vi "Main.vi"() -> ()   [LabVIEW 2023]
doc: "This template is for the Queued Message Handler design pattern.\n\nThe Event Handling Loop generates messages based on user interface actions.\n\nThe Message Handling Loop processes messages generated by the Event Handling Loop, or by other messages. The messages are string values, so new messages can be added easily to the Message Cases case structure in the Message Handling Loop. Each message cluster can also provide an optional value for Message Data, which is a variant that can be converted to whatever message-specific data is required."
uses:
  <extravilib>/ChannelInstances/Messenger-t'Message Queue.lvlib-Message Cluster.ctl'/Instantiate.vi
  <vilib>/Utility/error.llb/Error Cluster From Error Code.vi
  <extravilib>/ChannelInstances/Event Messenger-bool/))Channel.vi
  <extravilib>/ChannelInstances/Event Messenger-bool/Instantiate.vi
  <vilib>/ErrorRing/Error Ring.xnode
  <extravilib>/ChannelInstances/Event Messenger-bool.lvlib
  support/Message Queue/Message Queue.lvlib
panel:
  out "Loop Iteration Time":u32
  out "Create Data Time":u32
  out "ITER":i32
  out "Intensity Graph":u8[][](graph)
  in  "Start Parallel":bool
  in  "Exit":bool
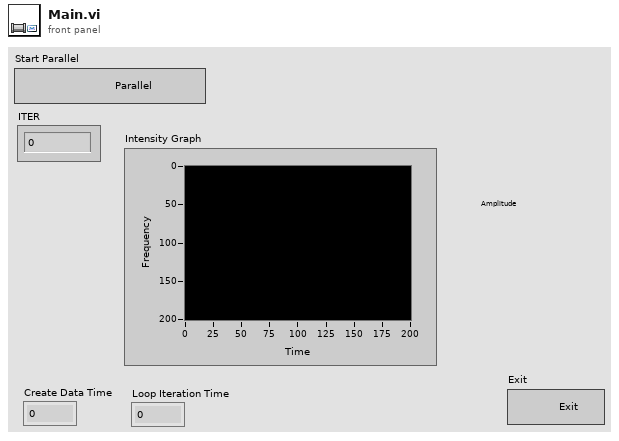
[diagram p1: front panel]
types:
  T1 = typedef "Messenger-t'Message Queue.lvlib-Message Cluster.ctl'.lvlib/))Channel.ctl" = refnum<queue>
  T2 = typedef "Event Messenger-bool.lvlib/))Channel.ctl" = refnum<queue>
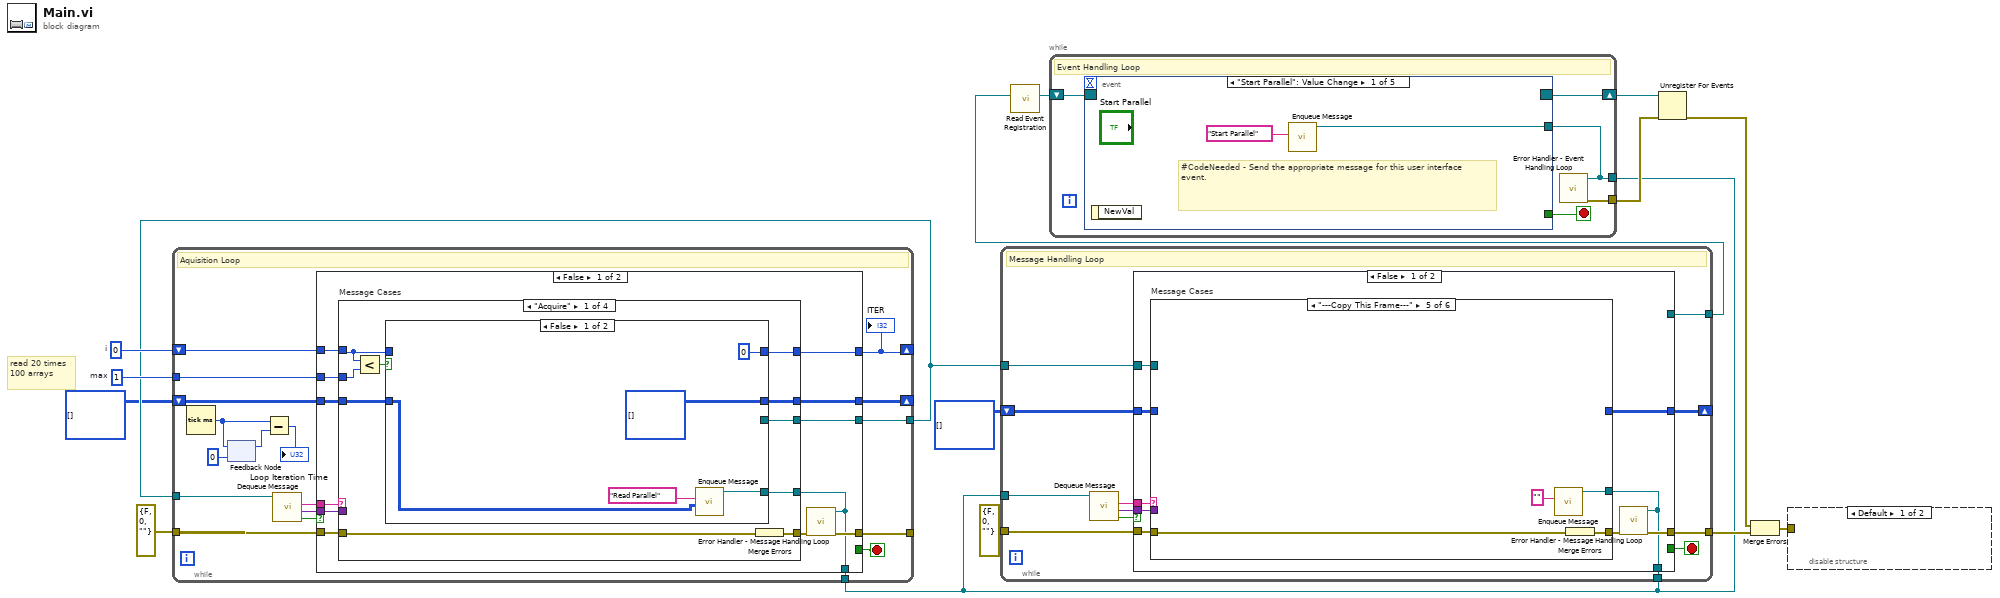
[diagram p0: block diagram]
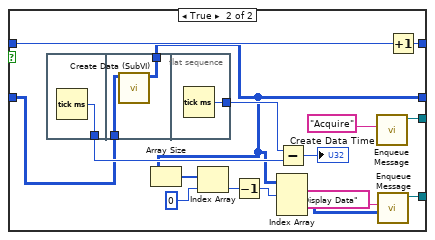
[diagram p2: hidden frame]
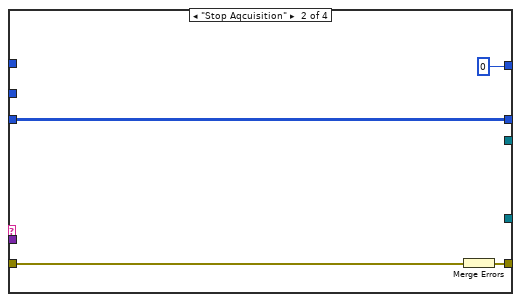
[diagram p3: hidden frame]
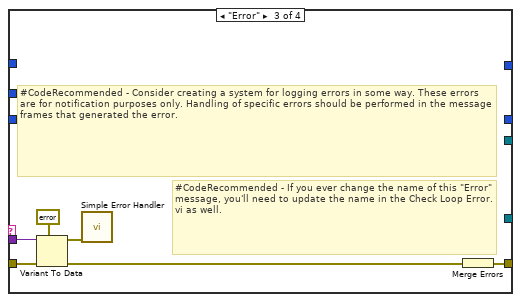
[diagram p4: hidden frame]
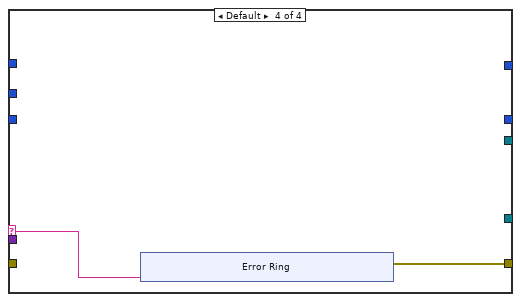
[diagram p5: hidden frame]
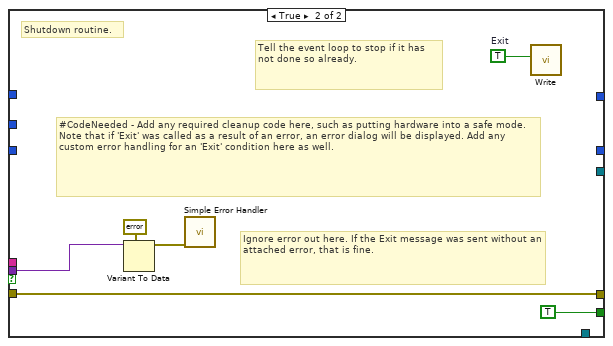
[diagram p6: hidden frame]
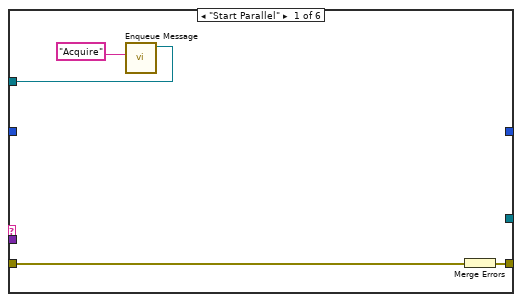
[diagram p7: hidden frame]
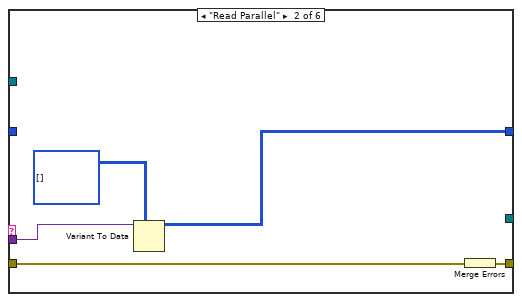
[diagram p8: hidden frame]
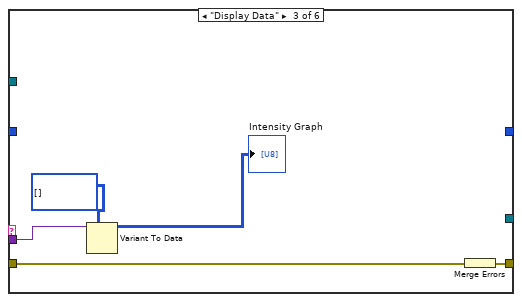
[diagram p9: hidden frame]
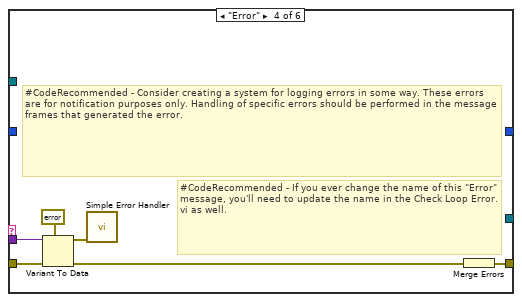
[diagram p10: hidden frame]
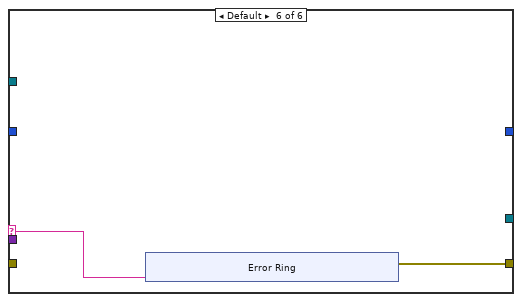
[diagram p11: hidden frame]
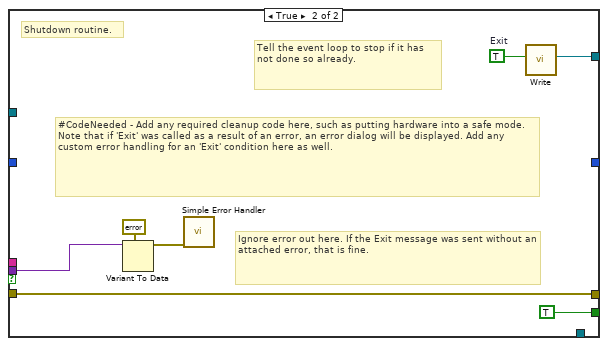
[diagram p12: hidden frame]
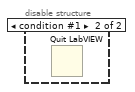
[diagram p13: hidden frame]
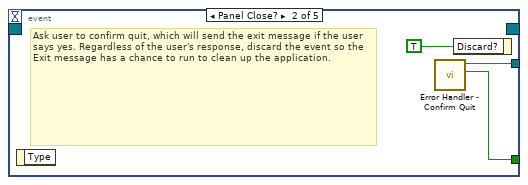
[diagram p14: hidden frame]
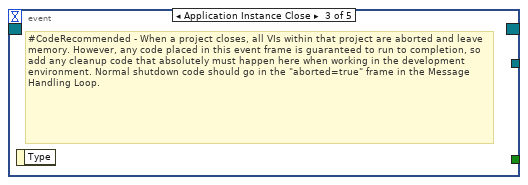
[diagram p15: hidden frame]
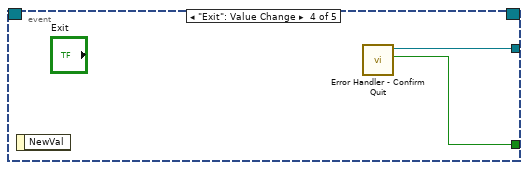
[diagram p16: hidden frame]
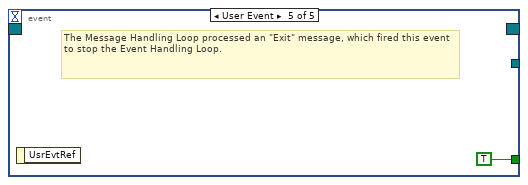
[diagram p17: hidden frame]
diagram:
  w4 = 0  # i
  w5 = 1  # max
  # "read 20 times\n100 arrays"
  n1 = while {
    tunnel: [w32] -> _
    tunnel: w3 -> [w29]
    tunnel: errorcluster {"status"=FALSE, "code"=0, "source"=""} ("error IO") -> [w31]
    tunnel: [w30] -> w6
    tunnel: w5 -> [w25]
    shift-right: [w23] -> _
    shift-left: w4 -> [w24]
    tunnel: [w22] -> w3
    shift-right: [w17] -> _
    shift-left: u8[][][] [] ("element") -> [w16]
    stop <- w33 stop-if-true
    # "Aquisition Loop"
    n2 = Tick Count (ms)() -> (millisecond timer value=w19:u32)
    n3 = feedback-in #1(w19) -> ()
    n4 = feedback #1(u32 0 ("millisecond timer value")) -> (w20:u32)
    n5 = Subtract(x=w19, y=w20) -> (x-y=→"Loop Iteration Time":u32)
    n6 = call "Dequeue Message.vi"("channel"=w29) -> ("channel aborted"=w26:bool, "message data"=w27:variant, "message"=w28:string)  [unwired: 8 in]
    n7 = case shown="False" w26 {
      tunnel: [_ TRUE] -> w33
      tunnel: [w45 w104] -> w32
      tunnel: w28 -> [w43 _]
      tunnel: w27 -> [w42 w101]
      tunnel: w31 -> [w41 w104]
      tunnel: [w40 _] -> w30
      tunnel: w25 -> [w39 _]
      tunnel: w24 -> [w38 _]
      tunnel: [w37 _] -> w23
      tunnel: [w36 _] -> w22
      tunnel: w16 -> [w35 _]
      tunnel: [w34 _] -> w17
      frame False {
        n8 = case "Message Cases" shown="\"Acquire\"" w43 {
          selector: w43 -> [_ _ _ w91]
          tunnel: w41 -> [w54 w83 w90 _]
          tunnel: [w55 w84 w85 w92] -> w44
          tunnel: w42 -> [_ _ w89 _]
          tunnel: [w53 _ _ _] -> w40
          tunnel: w39 -> [w49 _ _ _]
          tunnel: w38 -> [w50 _ _ _]
          tunnel: [w52 0 _ _] -> w37
          tunnel: [w48 _ _ _] -> w36
          tunnel: w35 -> [w47 w81 _ _]
          tunnel: [w46 w81 _ _] -> w34
          frame "Acquire" {
            # "Something - Replace this message with functionality for your own application."
            n9 = Less?(x=w50, y=w49) -> (x < y?=w51:bool)
            n10 = case shown="False" w51 {
              tunnel: [w58 w76] -> w53
              tunnel: [0 w74] -> w52
              tunnel: w50 -> [_ w73]
              tunnel: [_ w71] -> w48
              tunnel: w47 -> [w56 w67]
              tunnel: [u8[][][] [] ("element") w62] -> w46
              frame False {
                n11 = call "Enqueue Message.vi"("data (empty)"=w56, "message"="Read Parallel") -> ("channel"=w58:T1)  [unwired: 9 in]
              }
              frame True {
                n12 = flat-sequence {
                  tunnel: [w77] -> w69
                  tunnel: w67 -> [w78]
                  tunnel: [w79] -> w62
                  tunnel: [w80] -> w70
                  frame #0 {
                    n13 = Tick Count (ms)() -> (millisecond timer value=w77:u32)
                  }
                  frame #1 {
                    n14 = call "Create Data (SubVI).vi"("appended array"=w78) -> ("appended array 2"=w79:u8[][][])  [unwired: 10 in]
                  }
                  frame #2 {
                    n15 = Tick Count (ms)() -> (millisecond timer value=w80:u32)
                  }
                }
                n16 = Array Size(array=w62) -> (size(s)=w66:i32[])
                n17 = Index Array(array=w66, index=0) -> (element=w64:i32)
                n18 = Decrement(x=w64) -> (x-1=w63:i32)
                n19 = Index Array(array=w62, index (dim 0)=w63) -> (element=w61:u8[][])  [unwired: 2 in]
                n20 = Subtract(x=w70, y=w69) -> (x-y=→"Create Data Time":u32)
                n21 = call "Enqueue Message.vi"("message"="Acquire") -> ("channel"=w71:T1)  [unwired: 10 in]
                n22 = call "Enqueue Message.vi"("data (empty)"=w61, "message"="Display Data") -> ("channel"=w76:T1)  [unwired: 9 in]
                n23 = Increment(x=w73) -> (x+1=w74:i32)
              }
            }
            n24 = Merge Errors(w54) -> (w55:errorcluster)
          }
          frame "Stop Aqcuisition" {
            # "Something - Replace this message with functionality for your own application."
            n25 = Merge Errors(w83) -> (w84:errorcluster)
          }
          frame "Error" {
            # "#CodeRecommended - If you ever change the name of this \"Error\" message, you'll need to update the name in the Check Loop Error.vi as well."
            # "#CodeRecommended - Consider creating a system for logging errors in some way. These errors are for notification purposes only. Handling of specific errors should be performed in the message frames that generated the error."
            # "Error - Display an error dialog. This message is sent by the \"Error Handler\" VIs at the end of other loops in this application."
            n26 = Variant To Data(error in=w90, type=errorcluster {"status"=FALSE, "code"=0, "source"=""} ("error constant"), Variant=w89) -> (data=w87:errorcluster, error out=w86:errorcluster)
            n27 = call <vilib>:"Simple Error Handler.vi"("error in (no error)"=w87) -> ()  [unwired: 4 in, 5 out]
            n28 = Merge Errors(w86) -> (w85:errorcluster)
          }
          frame Default {
            # "'Default' case only runs if there is a message that isn't defined in any of the other cases.  Output a programming error."
            n29 = xnode "Error Ring"("parameter 0"=w91) -> ("error out"=w92:errorcluster)
          }
        }
        n30 = call "Error Handler - Message Handling Loop.vi"("channel"=w40, "error in (no error)"=w44) -> ("dup error in"=w45:errorcluster)  [unwired: 9 in]
      }
      frame True {
        w100 = TRUE  # Exit
        # "Tell the event loop to stop if it has not done so already."
        # "Ignore error out here. If the Exit message was sent without an attached error, that is fine."
        # "#CodeNeeded - Add any required cleanup code here, such as putting hardware into a safe mode. Note that if 'Exit' was called as a result of an error, an error dialog will be displayed. Add any custom error handling for an 'Exit' condition here as well."
        # "Shutdown routine."
        n31 = Variant To Data(type=errorcluster {"status"=FALSE, "code"=0, "source"=""} ("error constant"), Variant=w101) -> (data=w102:errorcluster)  [unwired: 1 in, 1 out]
        n32 = call <vilib>:"Simple Error Handler.vi"("error in (no error)"=w102) -> ()  [unwired: 4 in, 5 out]
        n33 = call <extravilib>:"Write.vi"("element"=w100) -> ()  [unwired: 9 in, 2 out]
      }
    }
    "ITER" <- w23
  }
  n34 = while {
    tunnel: [w116] -> w15
    tunnel: [w115] -> w11
    tunnel: w6 -> [w112]
    tunnel: errorcluster {"status"=FALSE, "code"=0, "source"=""} ("error IO") -> [w114]
    tunnel: w6 -> [w113]
    tunnel: w3 -> [w108]
    shift-right: [w106] -> _
    shift-left: u8[][][] [] ("element") -> [w107]
    stop <- w117 stop-if-true
    # "Message Handling Loop"
    n35 = call "Dequeue Message.vi"("channel"=w112) -> ("channel aborted"=w109:bool, "message data"=w110:variant, "message"=w111:string)  [unwired: 8 in]
    n36 = case shown="False" w109 {
      tunnel: [_ TRUE] -> w117
      tunnel: [w126 w165] -> w116
      tunnel: [_ w160] -> w115
      tunnel: w111 -> [w124 _]
      tunnel: w110 -> [w123 w162]
      tunnel: w114 -> [w122 w165]
      tunnel: [w121 _] -> w113
      tunnel: [w120 _] -> w108
      tunnel: w107 -> [w119 _]
      tunnel: [w118 _] -> w106
      frame False {
        n37 = case "Message Cases" shown="\"---Copy This Frame---\"" w124 {
          selector: w124 -> [_ _ _ _ _ w151]
          tunnel: w122 -> [w129 w134 w139 w146 w150 _]
          tunnel: [w130 w135 w140 w141 w149 w152] -> w125
          tunnel: w123 -> [_ w133 w138 w145 _ _]
          tunnel: [_ _ _ _ w147 _] -> w121
          tunnel: [w127 _ _ _ _ _] -> w120
          tunnel: w119 -> [_ _ _ _ _ _]
          tunnel: [_ w131 _ _ _ _] -> w118
          frame "Start Parallel" {
            # "Something - Replace this message with functionality for your own application."
            n38 = call "Enqueue Message.vi"("message"="Acquire") -> ("channel"=w127:T1)  [unwired: 10 in]
            n39 = Merge Errors(w129) -> (w130:errorcluster)
          }
          frame "Read Parallel" {
            # "Something - Replace this message with functionality for your own application."
            n40 = Variant To Data(type=u8[][][] [] ("element"), Variant=w133) -> (data=w131:u8[][][])  [unwired: 1 in, 1 out]
            n41 = Merge Errors(w134) -> (w135:errorcluster)
          }
          frame "Display Data" {
            # "Something - Replace this message with functionality for your own application."
            n42 = Variant To Data(type=u8[][] [] ("element"), Variant=w138) -> (data=→"Intensity Graph":u8[][])  [unwired: 1 in, 1 out]
            n43 = Merge Errors(w139) -> (w140:errorcluster)
          }
          frame "Error" {
            # "#CodeRecommended - If you ever change the name of this \"Error\" message, you'll need to update the name in the Check Loop Error.vi as well."
            # "#CodeRecommended - Consider creating a system for logging errors in some way. These errors are for notification purposes only. Handling of specific errors should be performed in the message frames that generated the error."
            # "Error - Display an error dialog. This message is sent by the \"Error Handler\" VIs at the end of other loops in this application."
            n44 = Variant To Data(error in=w146, type=errorcluster {"status"=FALSE, "code"=0, "source"=""} ("error constant"), Variant=w145) -> (data=w143:errorcluster, error out=w142:errorcluster)
            n45 = call <vilib>:"Simple Error Handler.vi"("error in (no error)"=w143) -> ()  [unwired: 4 in, 5 out]
            n46 = Merge Errors(w142) -> (w141:errorcluster)
          }
          frame "---Copy This Frame---" {
            # "Duplicate this frame when creating new messages.  Change this comment in the duplicated frame to describe this message."
            n47 = call "Enqueue Message.vi"("message"="") -> ("channel"=w147:T1)  [unwired: 10 in]
            n48 = Merge Errors(w150) -> (w149:errorcluster)
          }
          frame Default {
            # "'Default' case only runs if there is a message that isn't defined in any of the other cases.  Output a programming error."
            n49 = xnode "Error Ring"("parameter 0"=w151) -> ("error out"=w152:errorcluster)
          }
        }
        n50 = call "Error Handler - Message Handling Loop.vi"("channel"=w121, "error in (no error)"=w125) -> ("dup error in"=w126:errorcluster)  [unwired: 9 in]
      }
      frame True {
        w161 = TRUE  # Exit
        # "Tell the event loop to stop if it has not done so already."
        # "Ignore error out here. If the Exit message was sent without an attached error, that is fine."
        # "#CodeNeeded - Add any required cleanup code here, such as putting hardware into a safe mode. Note that if 'Exit' was called as a result of an error, an error dialog will be displayed. Add any custom error handling for an 'Exit' condition here as well."
        # "Shutdown routine."
        n51 = Variant To Data(type=errorcluster {"status"=FALSE, "code"=0, "source"=""} ("error constant"), Variant=w162) -> (data=w163:errorcluster)  [unwired: 1 in, 1 out]
        n52 = call <vilib>:"Simple Error Handler.vi"("error in (no error)"=w163) -> ()  [unwired: 4 in, 5 out]
        n53 = call <extravilib>:"Write.vi"("element"=w161) -> ("channel"=w160:T2)  [unwired: 9 in, 1 out]
      }
    }
  }
  n54 = call <extravilib>:"Read Event Registration.vi"("channel"=w11) -> ("event registration refnum"=w10:refnum<event-registration>)  [unwired: 10 in]
  n55 = while {
    shift-right: [w170] -> w13
    shift-left: w10 -> [w171]
    tunnel: [w168] -> w12
    tunnel: w6 -> [w167]
    stop <- w169 stop-if-true
    # "Event Handling Loop"
    n56 = event shown="[0] \"Start Parallel\": Value Change" {
      selector: w171 -> [_ _ _ _ _]
      dyn-events: [_ _ _ _ _] -> w170
      timeout: _ -> [_ _ _ _ _]
      tunnel: [_ w174 _ w177 TRUE ("Discard?")] -> w169
      tunnel: [w173 w175 _ w178 _] -> w167
      event "Start Parallel": Value Change {
        # "#CodeNeeded - Send the appropriate message for this user interface event."
        n57 = event-data() -> ()  [unwired: 1 in, 1 out]
        n58 = call "Enqueue Message.vi"("message"="Start Parallel" ("Message")) -> ("channel"=w173:T1)  [unwired: 10 in]
      }
      event Panel Close? {
        # "Ask user to confirm quit, which will send the exit message if the user says yes. Regardless of the user's response, discard the event so the Exit message has a chance to run to clean up the application."
        n59 = event-data() -> ()  [unwired: 1 in, 1 out]
        n60 = call "Error Handler - Confirm Quit.vi"() -> ("exit confirmed"=w174:bool, "channel"=w175:T1)  [unwired: 10 in]
        n61 = event-data("Discard?"=TRUE) -> ()  [unwired: 1 in, 1 out]
      }
      event Application Instance Close {
        # "#CodeRecommended - When a project closes, all VIs within that project are aborted and leave memory. However, any code placed in this event frame is guaranteed to run to completion, so add any cleanup code that absolutely must happen here when working in the development environment. Normal shutdown code should go in the \"aborted=true\" frame in the Message Handling Loop."
        n62 = event-data() -> ()  [unwired: 1 in, 1 out]
      }
      event "Exit": Value Change {
        n63 = event-data() -> ()  [unwired: 1 in, 1 out]
        n64 = call "Error Handler - Confirm Quit.vi"() -> ("exit confirmed"=w177:bool, "channel"=w178:T1)  [unwired: 10 in]
      }
      event User Event {
        # "The Message Handling Loop processed an \"Exit\" message, which fired this event to stop the Event Handling Loop."
        n65 = event-data() -> ()  [unwired: 1 in, 1 out]
      }
    }
    n66 = call "Error Handler - Event Handling Loop.vi"("channel"=w167) -> ("dup error in"=w168:errorcluster)  [unwired: 10 in]
  }
  n67 = Unregister For Events(event registration refnum=w13, error in=w12) -> (error out=w14:errorcluster)
  n68 = Merge Errors(w14, w15) -> (w9:errorcluster)
  n69 = disable-structure shown="Default" {
    disable-tunnel: w9 -> [_ _]
    frame condition #0 (active) {
    }
    frame condition #1 {
      n70 = Quit LabVIEW() -> ()  [unwired: 1 in]
    }
  }
